vi "GHV232 CRAB Set Programs.vi"(6 "?":bool, 7 "HV on":bool, 8 "error in (no error)":errorcluster, 9 "I prog":sgl min=0 max=100 step=0.1, 10 "V prog":sgl min=0 max=100 step=0.1, 11 "VISA resource name":refnum<visa-resource-name>) -> (0 "error out":errorcluster, 3 "VISA resource name 2":refnum<visa-resource-name>)   [LabVIEW 2017]
panel:
  # "This VI formats the programs and enable signals\ninto an ASCII string and sends it to the power\nsupply."
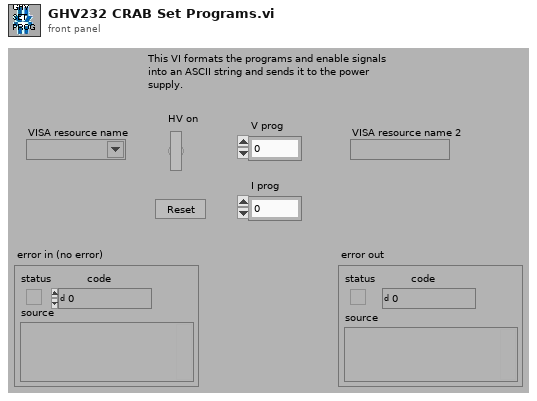
[diagram p1: front panel]
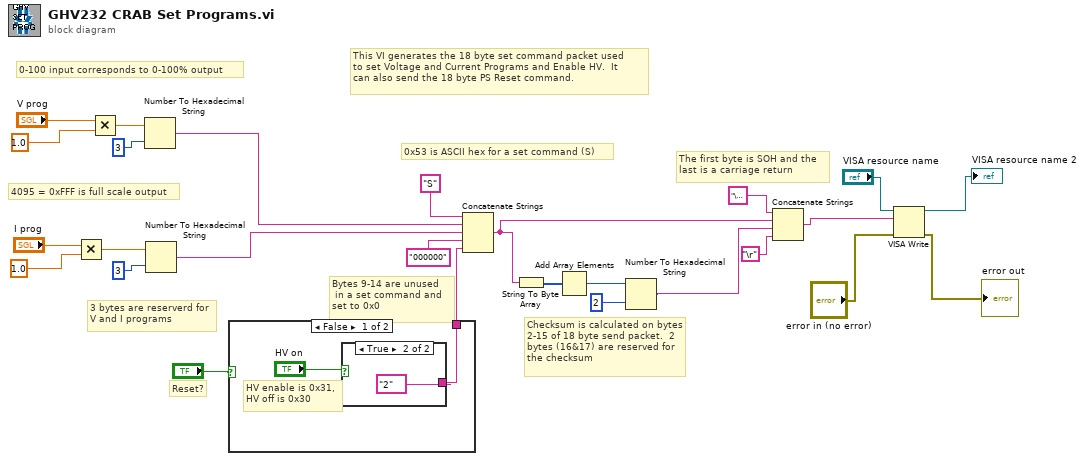
[diagram p0: block diagram]
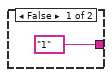
[diagram p2: hidden frame]
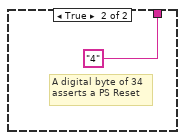
[diagram p3: hidden frame]
diagram:
  # "Reset?"
  # "This VI generates the 18 byte set command packet used \nto set Voltage and Current Programs and Enable HV.  It \ncan also send the 18 byte PS Reset command."
  # "The first byte is SOH and the\nlast is a carriage return"
  # "Bytes 9-14 are unused\n in a set command and\nset to 0x0"
  # "0x53 is ASCII hex for a set command (S)"
  # "Checksum is calculated on bytes 2-15 of 18 byte send packet.  2 bytes (16&17) are reserved for\nthe checksum"
  # "3 bytes are reserverd for\nV and I programs"
  # "4095 = 0xFFF is full scale output"
  # "0-100 input corresponds to 0-100% output"
  n1 = Multiply(x="I prog", y=1.0) -> (x*y=w21:dbl)
  n2 = Multiply(x="V prog", y=1.0) -> (x*y=w24:dbl)
  n3 = Number To Hexadecimal String(1:3, 2:w24) -> (0:w12:string)
  n4 = Number To Hexadecimal String(1:3, 2:w21) -> (0:w11:string)
  n5 = case shown="False" "?" {
    tunnel: [w27 "4"] -> w15
    frame False {
      # "HV enable is 0x31,\nHV off is 0x30"
      n6 = case shown="True" "HV on" {
        tunnel: ["1" "2"] -> w27
        frame False {
        }
        frame True {
        }
      }
    }
    frame True {
      # "A digital byte of 34\nasserts a PS Reset"
    }
  }
  n7 = Concatenate Strings("S", w12, w11, "000000", w15) -> (w14:string)
  n8 = String To Byte Array(string=w14) -> (unsigned byte array=w16:u8[])
  n9 = Add Array Elements(numeric array=w16) -> (sum=w9:u8)
  n10 = Number To Hexadecimal String(1:2, 2:w9) -> (0:w7:string)
  n11 = Concatenate Strings("\u0001", w14, w7, "\r") -> (w6:string)
  n12 = VISA Write(VISA resource name="VISA resource name", write buffer=w6, error in (no error)="error in (no error)") -> (VISA resource name out=→"VISA resource name 2":refnum<visa-resource-name>, error out=→"error out":errorcluster)  [unwired: 1 out]
